vi "CameraSetProperties.vi"(8 "error in (no error)":errorcluster, 10 "set?":bool, 11 "IMAQdx in":refnum<class "IMAQdx.lvclass">) -> (0 "error out":errorcluster, 2 "cam_params":cluster{"String":string, "value":variant}[](array[cluster]) caption="parameters", 3 "IMAQdx out":refnum<class "IMAQdx.lvclass">)   [LabVIEW 2010, in "IMAQdx.lvclass"]
uses:
  IMAQdx.lvclass
  <vilib>/vision/driver/IMAQdx.llb/IMAQdx Acquisition Mode.ctl
  IMAQdx.lvclass/IMAQdx.ctl
  Program Files (x86)/National Instruments/LabVIEW 2010/resource/objmgr/imaqdx.rc
  <vilib>/vision/driver/NI_Vision_Acquisition_Software.lvlib
panel:
  in  "cancel":bool
  in  "ok":bool
  in  "properties":enum32{"Page 2"}(tab)
  in  "TriggerSource":u32(ring) items=["Freerun"=0, "Line1"=1, "Line2"=2, "FixedRate"=5, "Software"=6]
  in  "Timeout":i32 min=0 step=1
  in  "ShiftPixelBits":bool
  in  "PixelFormat":u32(ring) items=["Mono8"=17301505, "Mono12"=17825797, "Mono12Packed"=17563654, "Mono14"=17825829]
  # "Camera Configuration"
  # "Remember, all settings and defaults can be configured in MAX"
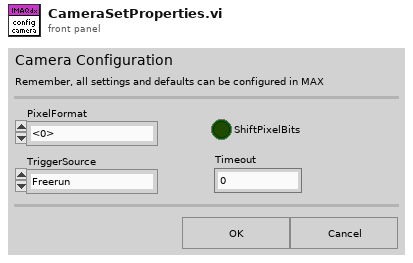
[diagram p1: front panel]
types:
  T1 = typedef "NI_Vision_Acquisition_Software.lvlib/IMAQdx Acquisition Mode.ctl" = enum32{"One Shot", "Continuous"}
  T2 = typedef "IMAQdx.ctl" = refnum<k21>
  T3 = enum8{"Enabled", "Disabled", "Disabled and Grayed Out"}
  T4 = typedef "Type Descriptor Enumeration__ogtk.ctl" = enum8{"<Null>", "I8", "I16", "I32", "I64", "U8", "U16", "U32", "U64", "SGL", "DBL", "EXT", "CSG", "CDB", "CXT", "0x0F", "0x10", "0x11", "0x12", "0x13", "0x14", "Enum U8", "Enum U16", "Enum U32", "Enum U64", "SGL PQ", "DBL PQ", "EXT PQ", "CSG PQ", "CDB PQ", "CXT PQ", "0x1F", "0x20", "Boolean", "0x22", "0x23", "0x24", "0x25", "0x26", "0x27", "0x28", "0x29", "0x2A", "0x2B", "0x2C", "0x2D", "0x2E", "0x2F", "String", "0x31", "Path", "Pict", "0x34", "0x35", "0x36", "DAQ", "0x38", "0x39", "0x3A", "0x3B", "0x3C", "0x3D", "0x3E", "0x3F", "Array", "0x41", "0x42", "0x43", "0x44", "0x45", "0x46", "0x47", "0x48", "0x49", "0x4A", "0x4B", "0x4C", "0x4D", "0x4E", "0x4F", "Cluster", "0x51", "0x52", "Variant", "Waveform", "0x55", "0x56", "0x57", "0x58", "0x59", "0x5A", "0x5B", "0x5C", "0x5D", "0x5E", "0x5F", "0x60", "0x61", "0x62", "0x63", "0x64", "0x65", "0x66", "0x67", "0x68", "0x69", "0x6A", "0x6B", "0x6C", "0x6D", "0x6E", "0x6F", "Refnum"}
  T5 = cluster{"Label.Text":string, "Variant":variant}[]
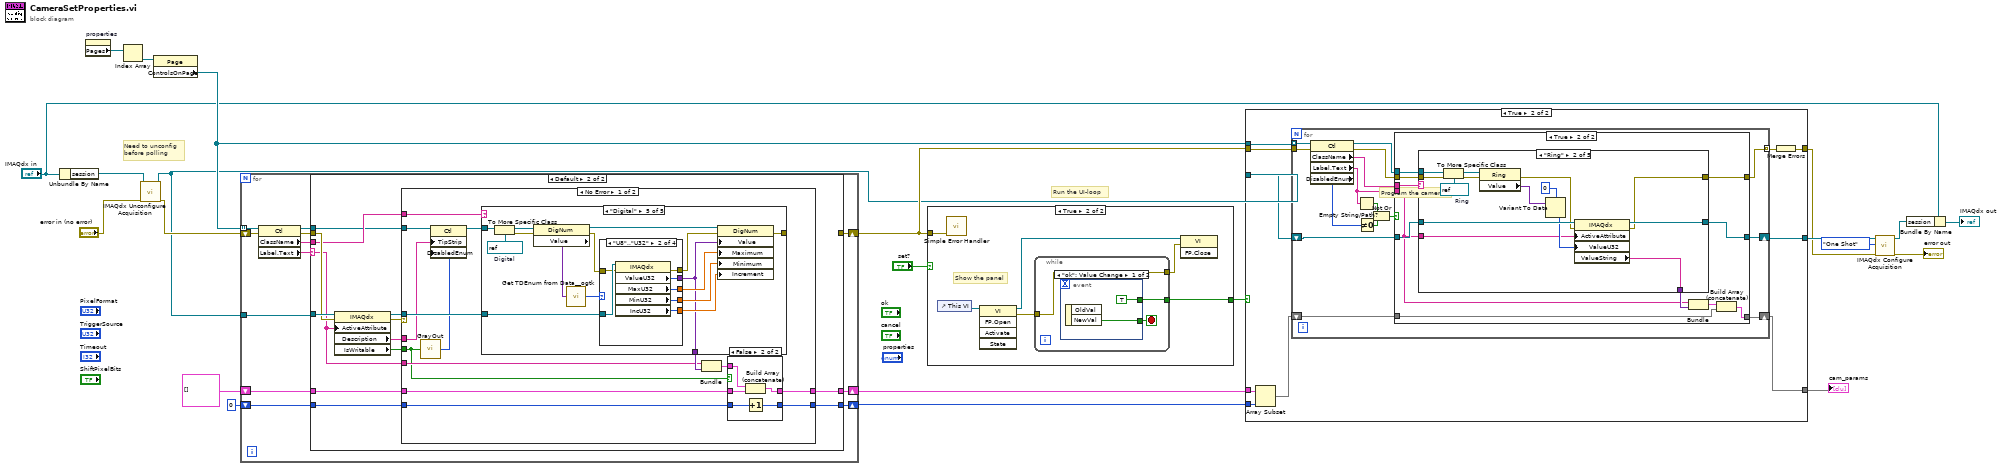
[diagram p0: block diagram]
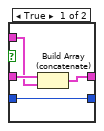
[diagram p3: hidden frame]
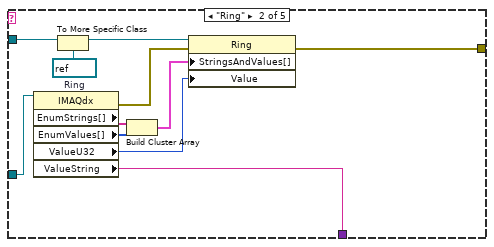
[diagram p5: hidden frame]
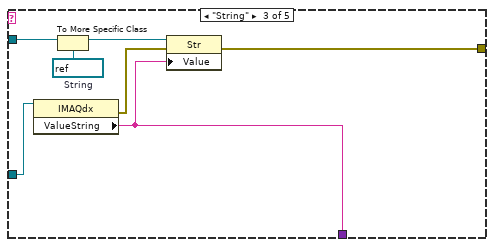
[diagram p6: hidden frame]
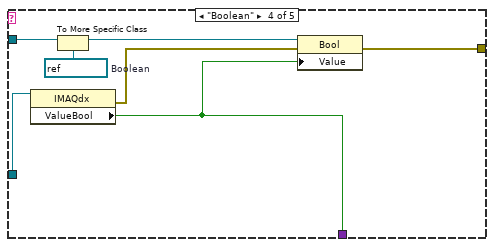
[diagram p7: hidden frame]
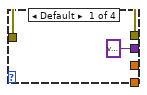
[diagram p8: hidden frame]
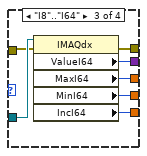
[diagram p9: hidden frame]
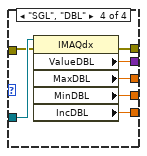
[diagram p10: hidden frame]
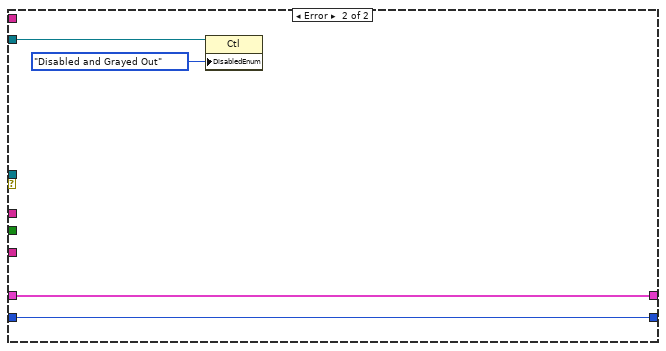
[diagram p11: hidden frame]
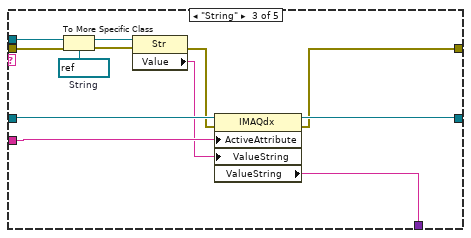
[diagram p15: hidden frame]
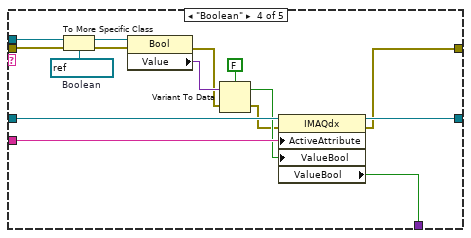
[diagram p16: hidden frame]
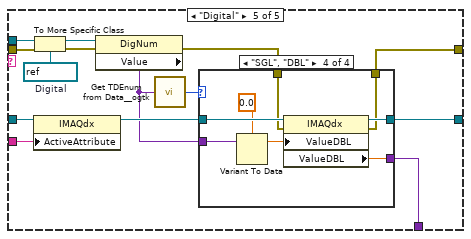
[diagram p17: hidden frame]
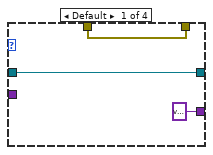
[diagram p18: hidden frame]
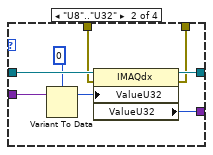
[diagram p19: hidden frame]
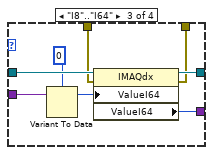
[diagram p20: hidden frame]
diagram:
  # "Need to unconfig\nbefore polling"
  # "Program the camera"
  # "Run the UI-loop"
  n1 = Unbundle By Name("IMAQdx in") -> ("session"=w17:refnum<k21>)
  n2 = property on="properties" class="TabCtl (strict)"() -> ("Pages"=w19:refnum<vi>[])  [unwired: 2 in, 2 out]
  n3 = Index Array(array=w19) -> (element=w20:refnum<vi>)  [unwired: 1 in]
  n4 = call <vilib>:"IMAQdx Unconfigure Acquisition.vi"("error in"="error in (no error)", "Session In"=w17) -> ("error out"=w12:errorcluster, "Session Out"=w6:T2)  [unwired: 8 in]
  n5 = property class="Page"(reference=w20) -> ("ControlsOnPage"=w18:refnum<vi>[])  [unwired: 1 in, 2 out]
  n6 = for {
    tunnel: w18 -> [w31] mode=indexing
    shift-right: [w34] -> w15
    shift-left: w12 -> [w28]
    shift-right: [w25] -> w7
    shift-left: cluster{string, "Variant":variant}[] [] -> [w26]
    tunnel: w6 -> [w33]
    shift-right: [w24] -> w4
    shift-left: 0 -> [w23]
    n7 = property class="Ctl"(reference=w31, error in=w28) -> (reference out=w30:refnum<vi>, error out=w32:errorcluster, "ClassName"=w29:string, "Label.Text"=w27:string)
    n8 = case shown="Default" w27 {
      selector: w27 -> [_ w46]
      tunnel: [w37 _] -> w34
      tunnel: w33 -> [_ w50]
      tunnel: w32 -> [w37 w49]
      tunnel: w30 -> [_ w42]
      tunnel: w29 -> [_ w47]
      tunnel: w26 -> [w36 w41]
      tunnel: [w36 w40] -> w25
      tunnel: [w35 w39] -> w24
      tunnel: w23 -> [w35 w38]
      frame "" {
      }
      frame Default {
        n9 = property class="IMAQdx"(reference=w50, error in=w49, "ActiveAttribute"=w46) -> (reference out=w48:T2, error out=w45:errorcluster, "Description"=w44:string, "IsWritable"=w43:bool)
        n10 = case shown="No Error" w45 {
          tunnel: w48 -> [w64 _]
          tunnel: w42 -> [w60 w139]
          tunnel: w47 -> [w63 _]
          tunnel: w46 -> [w61 _]
          tunnel: w44 -> [w58 _]
          tunnel: w43 -> [w56 _]
          tunnel: w41 -> [w55 w138]
          tunnel: [w53 w138] -> w40
          tunnel: [w52 w137] -> w39
          tunnel: w38 -> [w51 w137]
          frame No Error {
            n11 = call "GrayOut.vi"("enabled?"=w56) -> ("state"=w57:T3)
            n12 = property class="Ctl"(reference=w60, "TipStrip"=w58, "DisabledEnum"=w57) -> (reference out=w59:refnum<vi>)  [unwired: 1 in, 1 out]
            n13 = case shown="\"Digital\"" w63 {
              tunnel: w64 -> [_ w84 w91 w98 w113]
              tunnel: w59 -> [_ w81 w90 w97 w112]
              tunnel: [_ w76 w86 w93 w110] -> _
              tunnel: [_ w74 w85 w92 w99] -> w62
              frame Default {
              }
              frame "Ring" {
                w80 = refnum<vi> refnum  # Ring
                n14 = property class="IMAQdx"(reference=w84) -> (error out=w77:errorcluster, "EnumStrings[]"=w83:string[], "EnumValues[]"=w82:u32[], "ValueU32"=w75:u32, "ValueString"=w74:string)  [unwired: 1 in, 1 out]
                n15 = To More Specific Class(target class=w80, reference=w81) -> (specific class reference=w79:refnum<vi>)  [unwired: 1 in, 1 out]
                n16 = Build Cluster Array(w83, w82) -> (w78:cluster{string, u32}[])
                n17 = property class="Ring"(reference=w79, error in=w77, "StringsAndValues[]"=w78, "Value"=w75) -> (error out=w76:errorcluster)  [unwired: 1 out]
              }
              frame "String" {
                w89 = refnum<vi> refnum  # String
                n18 = property class="IMAQdx"(reference=w91) -> (error out=w87:errorcluster, "ValueString"=w85:string)  [unwired: 1 in, 1 out]
                n19 = To More Specific Class(target class=w89, reference=w90) -> (specific class reference=w88:refnum<vi>)  [unwired: 1 in, 1 out]
                n20 = property class="Str"(reference=w88, error in=w87, "Value"=w85) -> (error out=w86:errorcluster)  [unwired: 1 out]
              }
              frame "Boolean" {
                w96 = refnum<vi> refnum  # Boolean
                n21 = property class="IMAQdx"(reference=w98) -> (error out=w94:errorcluster, "ValueBool"=w92:bool)  [unwired: 1 in, 1 out]
                n22 = To More Specific Class(target class=w96, reference=w97) -> (specific class reference=w95:refnum<vi>)  [unwired: 1 in, 1 out]
                n23 = property class="Bool"(reference=w95, error in=w94, "Value"=w92) -> (error out=w93:errorcluster)  [unwired: 1 out]
              }
              frame "Digital" {
                w111 = refnum<vi> refnum  # Digital
                n24 = To More Specific Class(target class=w111, reference=w112) -> (specific class reference=w108:refnum<vi>, error out=w102:errorcluster)  [unwired: 1 in]
                n25 = property class="DigNum"(reference=w108, error in=w102) -> (reference out=w107:refnum<vi>, error out=w101:errorcluster, "Value"=w109:variant)
                n26 = call <userlib>:"Get TDEnum from Data__ogtk.vi"("Data"=w109) -> ("Type Descriptor Enumeration"=w106:T4)  [unwired: 4 in]
                n27 = case shown="\"U8\"..\"U32\"" w106 {
                  tunnel: w113 -> [_ w122 w129 w136]
                  tunnel: [variant ("Variant") w121 w128 w135] -> w99
                  tunnel: [_ w120 w125 w132] -> w105
                  tunnel: [_ w119 w126 w133] -> w104
                  tunnel: [_ w118 w127 w134] -> w103
                  tunnel: w101 -> [w114 w117 w124 w131]
                  tunnel: [w114 w116 w123 w130] -> w100
                  frame Default {
                  }
                  frame "U8".."U32" {
                    n28 = property class="IMAQdx"(reference=w122, error in=w117) -> (error out=w116:errorcluster, "ValueU32"=w121:u32, "MaxU32"=w118:u32, "MinU32"=w119:u32, "IncU32"=w120:u32)  [unwired: 1 out]
                  }
                  frame "I8".."I64" {
                    n29 = property class="IMAQdx"(reference=w129, error in=w124) -> (error out=w123:errorcluster, "ValueI64"=w128:i64, "MaxI64"=w127:i64, "MinI64"=w126:i64, "IncI64"=w125:i64)  [unwired: 1 out]
                  }
                  frame "SGL", "DBL" {
                    n30 = property class="IMAQdx"(reference=w136, error in=w131) -> (error out=w130:errorcluster, "ValueDBL"=w135:dbl, "MaxDBL"=w134:dbl, "MinDBL"=w133:dbl, "IncDBL"=w132:dbl)  [unwired: 1 out]
                  }
                }
                n31 = property class="DigNum"(reference=w107, error in=w100, "Value"=w99, "Maximum"=w103, "Minimum"=w104, "Increment"=w105) -> (error out=w110:errorcluster)  [unwired: 1 out]
              }
            }
            n32 = Bundle(w61, "Variant"=w62) -> (w54:cluster{string, "Variant":variant})  [unwired: 1 in]
            n33 = case shown="False" w56 {
              tunnel: w55 -> [w68 w71]
              tunnel: w54 -> [w67 w72]
              tunnel: [w66 w73] -> w53
              tunnel: [w65 w70] -> w52
              tunnel: w51 -> [w65 w69]
              frame True {
                n34 = Build Array (concatenate)(w68, w67) -> (w66:cluster{string, "Variant":variant}[])
              }
              frame False {
                n35 = Build Array (concatenate)(w72, w71) -> (w73:cluster{string, "Variant":variant}[])
                n36 = Increment(x=w69) -> (x+1=w70:i32)
              }
            }
          }
          frame Error {
            n37 = property class="Ctl"(reference=w139, "DisabledEnum"=T3."Disabled and Grayed Out" ("Disabled")) -> ()  [unwired: 1 in, 2 out]
          }
        }
      }
    }
  }
  n38 = case shown="True" "set?" {
    tunnel: [FALSE ("ok") w145] -> w22
    tunnel: w15 -> [_ w142]
    frame False {
    }
    frame True {
      # "Show the panel"
      n39 = control-ref of="This VI"() -> (w147:refnum<vi>)
      n40 = call <vilib>:"Simple Error Handler.vi"("error in (no error)"=w142) -> ()  [unwired: 4 in, 5 out]
      n41 = invoke class="VI" method="FP.Open"(reference=w147) -> (reference out=w143:refnum<vi>, error out=w146:errorcluster)  [unwired: 4 in, 3 out]
      n42 = while {
        tunnel: w146 -> [w148]
        tunnel: [w149] -> w145
        tunnel: [w148] -> w144
        stop <- w150 stop-if-true
        n43 = event shown="[0] \"ok\": Value Change" {
          selector: _ -> [_ _]
          dyn-events: _ -> [_ _]
          timeout: _ -> [_ _]
          tunnel: [w152 TRUE ("NewVal")] -> w150
          tunnel: [TRUE ("ok") _] -> w149
          event "ok": Value Change {
            n44 = event-data() -> ("NewVal"=w152:bool)  [unwired: 1 in, 1 out]
          }
          event "cancel": Value Change; Panel Close; Application Instance Close {
            n45 = event-data() -> ()  [unwired: 1 in, 2 out]
          }
        }
      }
      n46 = invoke class="VI" method="FP.Close"(reference=w143, error in=w144) -> ()  [unwired: 1 in, 3 out]
    }
  }
  n47 = case shown="True" w22 {
    tunnel: w18 -> [_ w166]
    tunnel: w6 -> [w154 w165]
    tunnel: w7 -> [w156 w160]
    tunnel: [w156 w164] -> w16
    tunnel: [w155 w157] -> w10
    tunnel: w15 -> [w155 w162]
    tunnel: [w154 w161] -> w11
    tunnel: w4 -> [_ w159]
    frame False {
    }
    frame True {
      n48 = Array Subset(array=w160, length=w159) -> (w158:cluster{string, "Variant":variant}[])  [unwired: 1 in]
      n49 = for {
        shift-right: [w177] -> w161
        shift-left: w165 -> [w180]
        shift-right: [w173] -> w164
        shift-left: w158 -> [w174]
        tunnel: w166 -> [w171] mode=indexing
        tunnel: w162 -> [w175]
        tunnel: [w181] -> w163 mode=indexing
        n50 = property class="Ctl"(reference=w171, error in=w175) -> (reference out=w178:refnum<vi>, error out=w179:errorcluster, "ClassName"=w176:string, "Label.Text"=w172:string, "DisabledEnum"=w170:T3)
        n51 = Empty String/Path?(string/path=w172) -> (empty?=w167:bool)
        n52 = Not Equal To 0?(x=w170) -> (x != 0?=w168:bool)
        n53 = Not Or(1:w168, 2:w167) -> (0:w169:bool)
        n54 = case shown="True" w169 {
          tunnel: [w183 w195] -> w181
          tunnel: w180 -> [w184 w186]
          tunnel: w179 -> [w183 w187]
          tunnel: w178 -> [_ w188]
          tunnel: [w184 w194] -> w177
          tunnel: w176 -> [_ w193]
          tunnel: w174 -> [w182 w190]
          tunnel: [w182 w189] -> w173
          tunnel: w172 -> [_ w185]
          frame False {
          }
          frame True {
            n55 = case shown="\"Ring\"" w193 {
              tunnel: w186 -> [w197 w211 w223 w238 w252]
              tunnel: w188 -> [_ w210 w222 w237 w251]
              tunnel: [w196 w198 w212 w224 w239] -> w195
              tunnel: [w197 w207 w219 w234 w249] -> w194
              tunnel: w187 -> [w196 w201 w215 w228 w246]
              tunnel: [_ w202 w216 w229 w241] -> w192
              tunnel: w185 -> [_ w203 w218 w233 w243]
              frame Default {
              }
              frame "Ring" {
                w209 = refnum<vi> refnum  # Ring
                n56 = To More Specific Class(target class=w209, reference=w210, error in=w201) -> (specific class reference=w208:refnum<vi>, error out=w200:errorcluster)
                n57 = property class="Ring"(reference=w208, error in=w200) -> (error out=w199:errorcluster, "Value"=w204:variant)  [unwired: 1 out]
                n58 = Variant To Data(Variant=w204, type=u32 0 ("ValueU32")) -> (data=w205:u32)  [unwired: 1 in, 1 out]
                n59 = property class="IMAQdx"(reference=w211, error in=w199, "ActiveAttribute"=w203, "ValueU32"=w205) -> (reference out=w207:T2, error out=w198:errorcluster, "ValueString"=w202:string)
              }
              frame "String" {
                w221 = refnum<vi> refnum  # String
                n60 = To More Specific Class(target class=w221, reference=w222, error in=w215) -> (specific class reference=w220:refnum<vi>, error out=w214:errorcluster)
                n61 = property class="Str"(reference=w220, error in=w214) -> (error out=w213:errorcluster, "Value"=w217:string)  [unwired: 1 out]
                n62 = property class="IMAQdx"(reference=w223, error in=w213, "ActiveAttribute"=w218, "ValueString"=w217) -> (reference out=w219:T2, error out=w212:errorcluster, "ValueString"=w216:string)
              }
              frame "Boolean" {
                w236 = refnum<vi> refnum  # Boolean
                n63 = To More Specific Class(target class=w236, reference=w237, error in=w228) -> (specific class reference=w235:refnum<vi>, error out=w227:errorcluster)
                n64 = property class="Bool"(reference=w235, error in=w227) -> (error out=w226:errorcluster, "Value"=w230:variant)  [unwired: 1 out]
                n65 = Variant To Data(error in=w226, Variant=w230, type=FALSE) -> (error out=w225:errorcluster, data=w231:bool)
                n66 = property class="IMAQdx"(reference=w238, error in=w225, "ActiveAttribute"=w233, "ValueBool"=w231) -> (reference out=w234:T2, error out=w224:errorcluster, "ValueBool"=w229:bool)
              }
              frame "Digital" {
                w250 = refnum<vi> refnum  # Digital
                n67 = property class="IMAQdx"(reference=w252, "ActiveAttribute"=w243) -> (reference out=w244:T2)  [unwired: 1 in, 1 out]
                n68 = To More Specific Class(target class=w250, reference=w251, error in=w246) -> (specific class reference=w248:refnum<vi>, error out=w245:errorcluster)
                n69 = property class="DigNum"(reference=w248, error in=w245) -> (error out=w240:errorcluster, "Value"=w242:variant)  [unwired: 1 out]
                n70 = call <userlib>:"Get TDEnum from Data__ogtk.vi"("Data"=w242) -> ("Type Descriptor Enumeration"=w247:T4)  [unwired: 4 in]
                n71 = case shown="\"SGL\", \"DBL\"" w247 {
                  tunnel: w244 -> [w255 w263 w271 w279]
                  tunnel: [w255 w262 w270 w278] -> w249
                  tunnel: w242 -> [_ w259 w267 w275]
                  tunnel: [variant ("Variant") w258 w266 w274] -> w241
                  tunnel: w240 -> [w253 w257 w264 w273]
                  tunnel: [w253 w256 w265 w272] -> w239
                  frame Default {
                  }
                  frame "U8".."U32" {
                    n72 = Variant To Data(Variant=w259, type=u32 0 ("ValueU32")) -> (data=w260:u32)  [unwired: 1 in, 1 out]
                    n73 = property class="IMAQdx"(reference=w263, error in=w257, "ValueU32"=w260) -> (reference out=w262:T2, error out=w256:errorcluster, "ValueU32"=w258:u32)
                  }
                  frame "I8".."I64" {
                    n74 = Variant To Data(Variant=w267, type=i64 0 ("ValueU32")) -> (data=w268:i64)  [unwired: 1 in, 1 out]
                    n75 = property class="IMAQdx"(reference=w271, error in=w264, "ValueI64"=w268) -> (reference out=w270:T2, error out=w265:errorcluster, "ValueI64"=w266:i64)
                  }
                  frame "SGL", "DBL" {
                    n76 = Variant To Data(Variant=w275, type=0.0 ("ValueU32")) -> (data=w276:dbl)  [unwired: 1 in, 1 out]
                    n77 = property class="IMAQdx"(reference=w279, error in=w273, "ValueDBL"=w276) -> (reference out=w278:T2, error out=w272:errorcluster, "ValueDBL"=w274:dbl)
                  }
                }
              }
            }
            n78 = Bundle("Label.Text"=w185, "Variant"=w192) -> (w191:cluster{"Label.Text":string, "Variant":variant})  [unwired: 1 in]
            n79 = Build Array (concatenate)(w191, w190) -> (w189:T5)
          }
        }
      }
      n80 = Merge Errors(w163) -> (w157:errorcluster)
    }
  }
  "cam_params" <- w16
  n81 = call <vilib>:"IMAQdx Configure Acquisition.vi"("error in"=w10, "Continuous?"=IMAQdx_Acquisition_Mode."One Shot", "Session In"=w11) -> ("error out"=→"error out":errorcluster, "Session Out"=w3:T2)  [unwired: 7 in]
  n82 = Bundle By Name(cluster="IMAQdx in", "session"=w3) -> (→"IMAQdx out":refnum<class "IMAQdx.lvclass">)
